vi "Setup for Test.vi"(11 "Application":refnum<class "Application.lvclass">) -> (0 "error out":errorcluster, 3 "Application":refnum<class "Application.lvclass">)   [LabVIEW 2017, in "Application.lvlib" / "Application.lvclass"]
uses:
  Application.lvclass
  Test Recipe/Class/Test Recipe.lvclass
  <vilib>/TSS/ACRObat Test Framework/Core Launcher/Core Manager Methods -- Enum.ctl
  <vilib>/TSS/ACRObat Test Framework/Core Launcher/Core Launcher.lvlib
  <vilib>/TSS/ACRObat Test Framework/Classes/Data/Data Repo/Class/Data Repo.lvclass
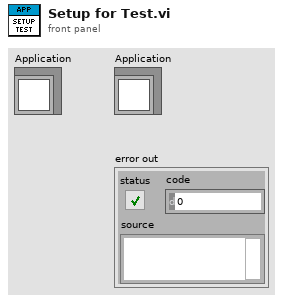
[diagram p1: front panel]
types:
  T1 = typedef "Core Launcher.lvlib/Core Manager Methods -- Enum.ctl" = enum16{"Spawn Objects", "Get Objects", "Destroy Objects"}
  T2 = typedef "Application.lvlib/App Properties.lvclass/Class Properties -- Cluster.ctl" = cluster{"UUT Info":T3[], "Test Information":refnum<vi>, "Gold Board":refnum<class "Golden Board.lvclass">, "Test Recipe":refnum<class "Test Recipe.lvclass">, "Instruments":refnum<class "Instrument.lvclass">[], "Mode":T4, "Test Results":T5[], "Station Config":refnum<class "Station Config.lvclass">, "Variable Engine":refnum<class "Variable Engine.lvclass">}
  T3 = typedef "Application.lvlib/App Properties.lvclass/UUT Reference -- Cluster.ctl" = cluster{"Serial Number Reference":refnum<vi>, "Status Message Reference":refnum<vi>}
  T4 = typedef "Application.lvlib/Application.lvclass/Op Mode -- Enum.ctl" = u16
  T5 = typedef "Application.lvlib/App Properties.lvclass/Test Result -- Cluster.ctl" = cluster{"Position":i32, "Pass":bool, "Fail Codes":string}
  T6 = typedef "Application.lvlib/Application.lvclass/Test Info -- Cluster.ctl" = cluster{"Time / Date":string, "Operator ID":string, "Material":string, "Log Field":string, "Test Time":string, "Software Revision":string}
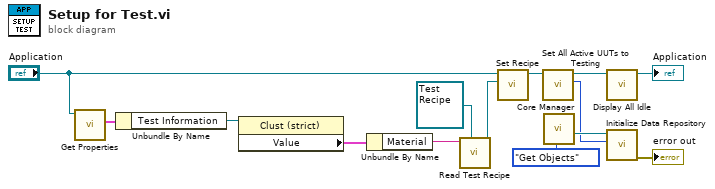
[diagram p0: block diagram]
diagram:
  n1 = call "Get Properties.vi"("Acrobat Template in"="Application") -> ("Class Properties"=w11:T2)  [unwired: 8 in, 2 out]
  n2 = Unbundle By Name(w11) -> ("Test Information"=w12:refnum<vi>)
  n3 = property class="Clust (strict)"(reference=w12) -> ("Value"=w13:T6)  [unwired: 1 in, 2 out]
  n4 = Unbundle By Name(w13) -> ("Material"=w14:string)
  n5 = call "Read Test Recipe.vi"("Test Recipe in"=refnum<class "Test Recipe.lvclass"> refnum ("Golden Board in"), "Material Type"=w14) -> ("Test Recipe out"=w9:refnum<class "Test Recipe.lvclass">)  [unwired: 8 in, 1 out]
  n6 = call "Set Recipe.vi"("Golden Board in"=w9, "Acrobat Template in"="Application") -> ("Acrobat Template out"=w5:refnum<class "Application.lvclass">)  [unwired: 8 in, 1 out]
  n7 = call "Set All Active UUTs to Testing.vi"("Application in"=w5) -> ("Number of Active DUTs"=w2:i32, "Application out"=w6:refnum<class "Application.lvclass">)  [unwired: 8 in, 1 out]
  n8 = call <vilib>:"Core Manager.vi"("Method"=Core_Manager_Methods_--_Enum."Get Objects") -> ("Data Repo"=w3:refnum<class "Data Repo.lvclass">)  [unwired: 6 in, 4 out]
  n9 = call "Display All Idle.vi"("Application in"=w6) -> ("Application out"=→"Application":refnum<class "Application.lvclass">)  [unwired: 9 in, 1 out]
  n10 = call <vilib>:"Initialize Data Repository.vi"("Number of DUTs"=w2, "Acrobat Template in"=w3) -> ("error out"=→"error out":errorcluster)  [unwired: 8 in, 1 out]
